vi "State Process.vi"(8 "error in (no error)":errorcluster, 11 "View Model":T1) -> (0 "error out":errorcluster, 3 "View Model":T1)   [LabVIEW 2017]
doc: "Process actual elevator controller state."
uses:
  View Model/Controls/View Model.ctl
  View Model/Controls/Shared Model.ctl
  Error Handler/Controls/Error Model.ctl
  Error Handler/Controls/Error Data.ctl
  Error Handler/Controls/Error Level.ctl
  Configuration/Controls/Config Model.ctl
  Configuration/Controls/Config Data Record.ctl
  Configuration/Controls/Config Command.ctl
  Controls/Control Model.ctl
  Controls/Elevator Location.ctl
  Controls/Elevator Status.ctl
  Controls/Control Event.ctl
  Controls/Control CMD.ctl
  Controls/Controller - Overhead.ctl
  Controls/Timer Commands.ctl
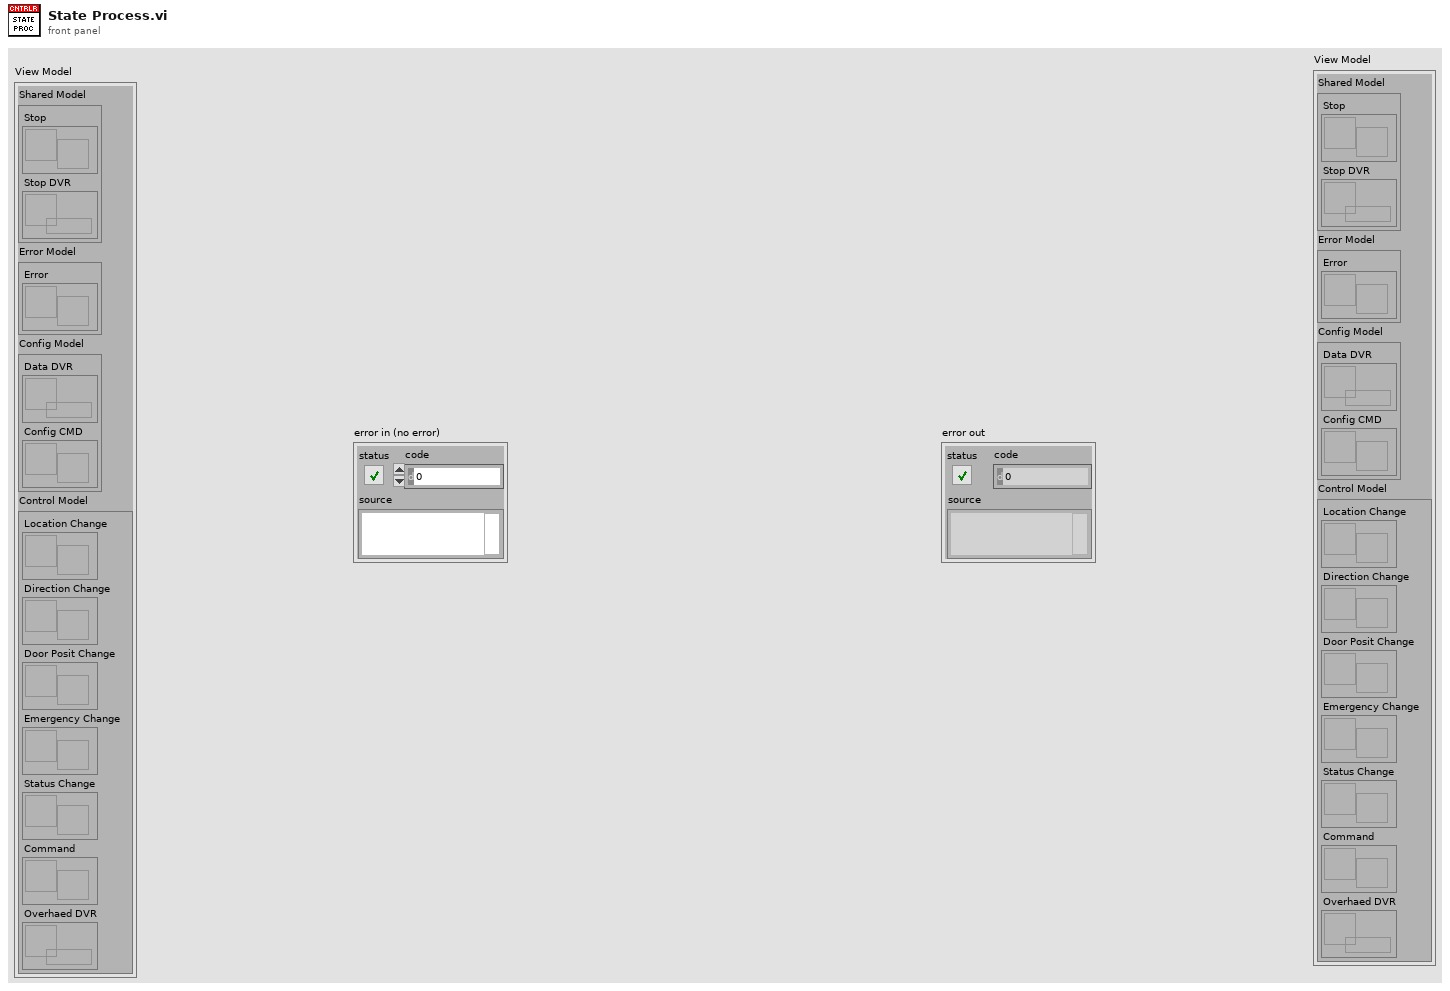
[diagram p1: front panel]
types:
  T1 = typedef "View Model.ctl" = cluster{"Shared Model":T2, "Error Model":T3, "Config Model":T4, "Control Model":T5}
  T2 = typedef "Shared Model.ctl" = cluster{"Stop":refnum<user-event>, "Stop DVR":refnum<data-value>}
  T3 = typedef "Error Model.ctl" = cluster{"Error":refnum<user-event>}
  T4 = typedef "Config Model.ctl" = cluster{"Data DVR":refnum<data-value>, "Config CMD":refnum<user-event>}
  T5 = typedef "Control Model.ctl" = cluster{"Location Change":refnum<user-event>, "Direction Change":refnum<user-event>, "Door Posit Change":refnum<user-event>, "Emergency Change":refnum<user-event>, "Status Change":refnum<user-event>, "Command":refnum<user-event>, "Overhaed DVR":refnum<data-value>}
  T6 = typedef "Elevator Status.ctl" = enum16{"No Request", "Initial", "Wait for 1st Request", "Start and Move", "Continue Move", "Analysis", "Stop at Floor", "Open/Close Door", "Emergency Call", "Terminate"}
  T7 = typedef "Timer Commands.ctl" = enum16{"Start", "Restart", "Get", "Pause"}
  T8 = typedef "Elevator Location.ctl" = enum16{"1st Floor", "2nd Floor", "3rd Floor", "4th Floor"}
  T9 = typedef "Control CMD.ctl" = enum16{"Idle", "Call", "Go Up", "Go Down", "Go to Floor", "Open Door", "Close Door", "Emergency"}
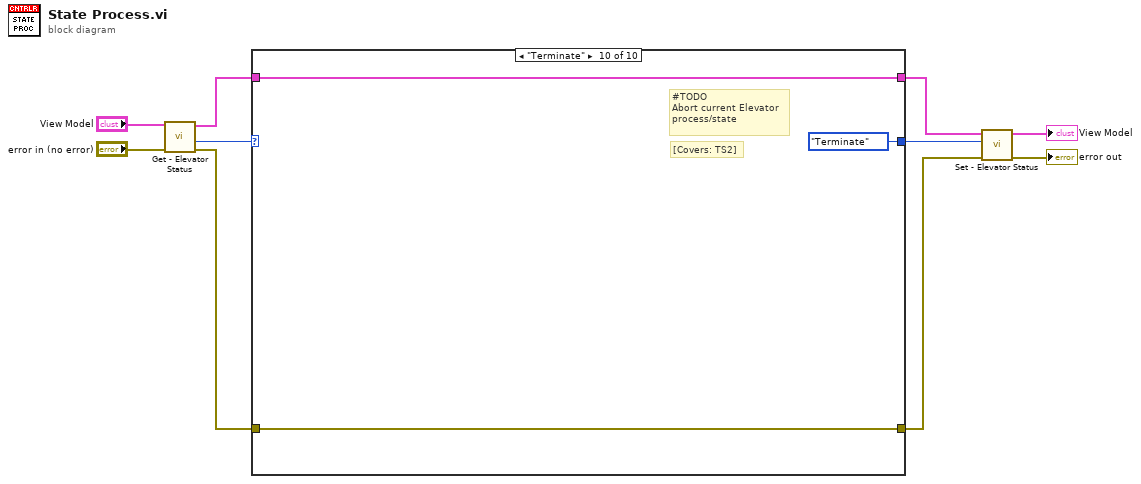
[diagram p0: block diagram]
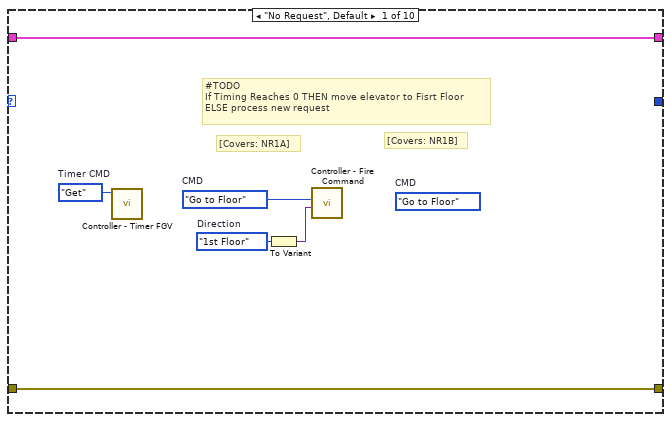
[diagram p2: hidden frame]
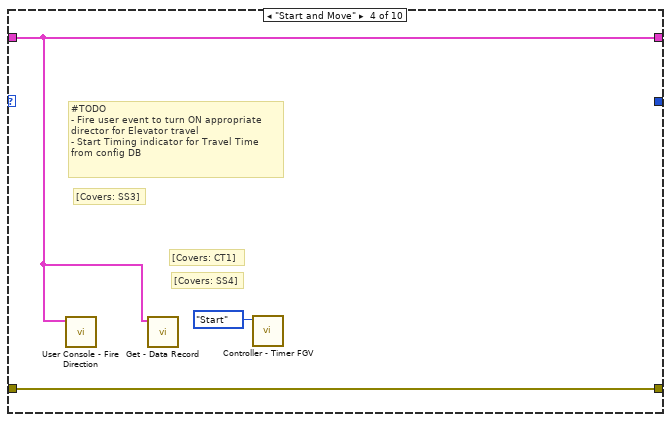
[diagram p5: hidden frame]
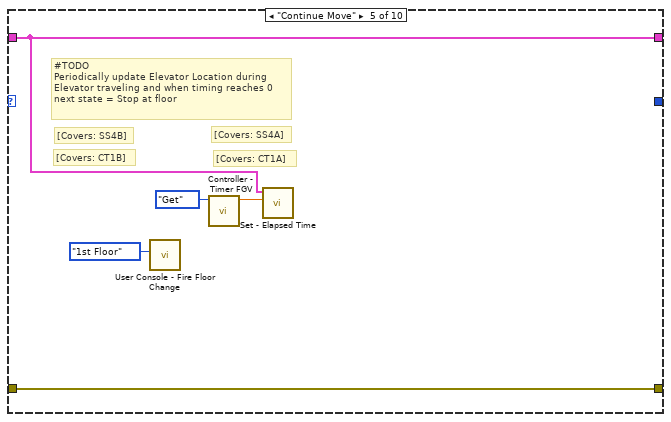
[diagram p6: hidden frame]
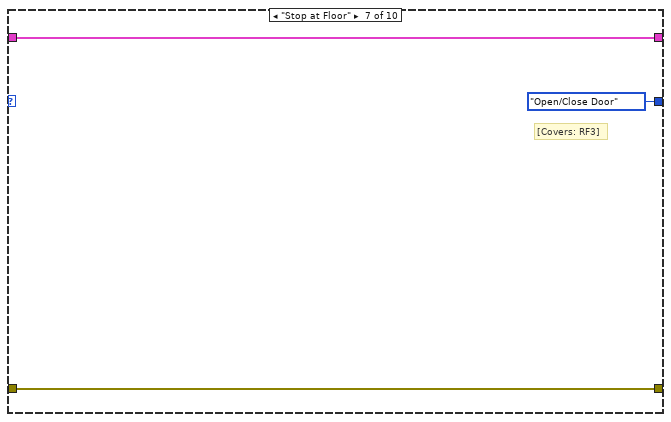
[diagram p8: hidden frame]
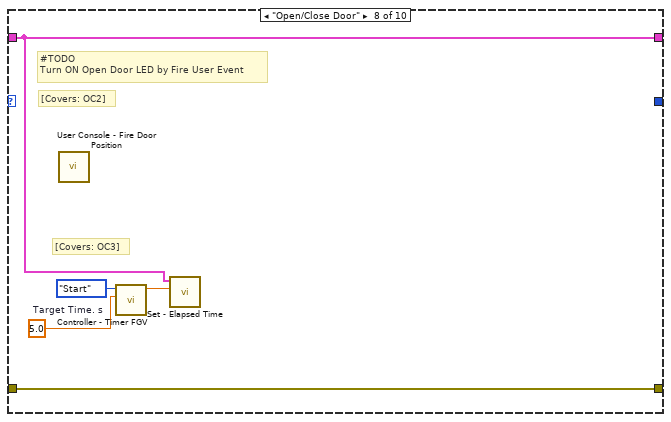
[diagram p9: hidden frame]
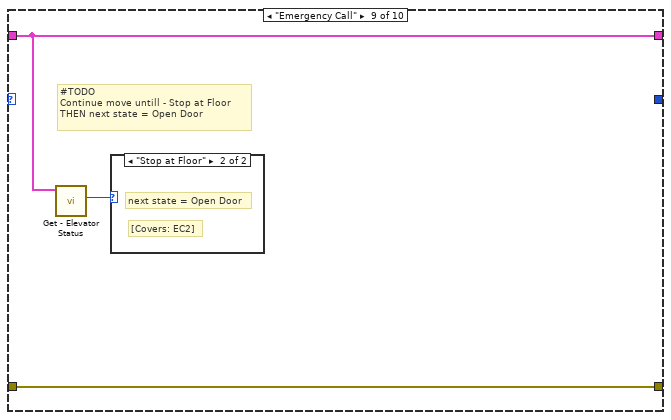
[diagram p10: hidden frame]
diagram:
  n1 = call "Get - Elevator Status.vi"("error in (no error)"="error in (no error)", "View Model"="View Model") -> ("error out"=w2:errorcluster, "Next Status"=w9:T6, "View Model"=w8:T1)  [unwired: 6 in, 1 out]
  n2 = case shown="\"Terminate\"" w9 {
    selector: w9 -> [_ w17 _ _ _ _ _ _ _ _]
    tunnel: w8 -> [w16 w19 w21 w22 w25 w31 w34 w36 w40 w45]
    tunnel: [w16 w19 w21 w22 w25 w31 w34 w36 w40 w45] -> w7
    tunnel: w2 -> [w15 w18 w20 w24 w29 w30 w33 w39 w42 w44]
    tunnel: [w15 w18 w20 w24 w29 w30 w33 w39 w42 w44] -> w3
    tunnel: [_ w17 _ _ _ _ Elevator_Status."Open/Close Door" ("Next Status") _ _ Elevator_Status."Terminate" ("Next Status")] -> w1
    frame "No Request", Default {
      (unwired) Control_CMD."Go to Floor"  # CMD
      w12 = Elevator_Location."1st Floor"  # Direction
      w13 = Control_CMD."Go to Floor"  # CMD
      w14 = Timer_Commands."Get"  # Timer CMD
      # "[Covers: NR1B]"
      # "[Covers: NR1A]"
      # "#TODO\nIf Timing Reaches 0 THEN move elevator to Fisrt Floor\nELSE process new request"
      n3 = call "Controller - Timer FGV.vi"("Timer CMD"=w14) -> ()  [unwired: 8 in, 3 out]
      n4 = To Variant(anything=w12) -> (Variant=w11:variant)
      n5 = call "Controller - Fire Command.vi"("Data"=w11, "CMD"=w13) -> ()  [unwired: 8 in, 2 out]
    }
    frame "Initial" {
    }
    frame "Wait for 1st Request" {
    }
    frame "Start and Move" {
      # "[Covers: CT1]"
      # "[Covers: SS4]"
      # "[Covers: SS3]"
      # "#TODO\n- Fire user event to turn ON appropriate \ndirector for Elevator travel\n- Start Timing indicator for Travel Time\nfrom config DB"
      n6 = call "User Console - Fire Direction.vi"("View Model"=w22) -> ()  [unwired: 9 in, 2 out]
      n7 = call "Get - Data Record.vi"("View Model"=w22) -> ()  [unwired: 8 in, 3 out]
      n8 = call "Controller - Timer FGV.vi"("Timer CMD"=Timer_Commands."Start") -> ()  [unwired: 8 in, 3 out]
    }
    frame "Continue Move" {
      # "[Covers: CT1B]"
      # "[Covers: CT1A]"
      # "[Covers: SS4B]"
      # "[Covers: SS4A]"
      # "#TODO\nPeriodically update Elevator Location during\nElevator traveling and when timing reaches 0\nnext state = Stop at floor"
      n9 = call "User Console - Fire Floor Change.vi"("Floor Selection"=Elevator_Location."1st Floor") -> ()  [unwired: 9 in, 2 out]
      n10 = call "Controller - Timer FGV.vi"("Timer CMD"=Timer_Commands."Get") -> ("Elapsed Time"=w26:dbl)  [unwired: 8 in, 2 out]
      n11 = call "Set - Elapsed Time.vi"("Elapsed Time"=w26, "View Model"=w25) -> ()  [unwired: 8 in, 2 out]
    }
    frame "Analysis" {
      # "[Covers: AS2C]"
      # "[Covers: AS2B]"
      # "[Covers: AS2A]"
      # "[Covers: AS2]"
      # "#TODO\nDetermines next ELevator states based on DVR values.\nIF the Elevator should stop on current floor THEN next state = Stop at Floor\nIF the Elevator should continue travel in current direction \n  THEN next state=Continue Move\nIF the Elevator changes direction THEN next state = Start and Move"
    }
    frame "Stop at Floor" {
      # "[Covers: RF3]"
    }
    frame "Open/Close Door" {
      w35 = 5.0  # Target Time. s
      # "[Covers: OC3]"
      # "[Covers: OC2]"
      # "#TODO\nTurn ON Open Door LED by Fire User Event"
      n12 = call "User Console - Fire Door Position.vi"() -> ()  [unwired: 10 in, 2 out]
      n13 = call "Controller - Timer FGV.vi"("Target Time. s"=w35, "Timer CMD"=Timer_Commands."Start") -> ("Elapsed Time"=w38:dbl)  [unwired: 7 in, 2 out]
      n14 = call "Set - Elapsed Time.vi"("Elapsed Time"=w38, "View Model"=w36) -> ()  [unwired: 8 in, 2 out]
    }
    frame "Emergency Call" {
      # "#TODO\nContinue move untill - Stop at Floor\nTHEN next state = Open Door"
      n15 = call "Get - Elevator Status.vi"("View Model"=w40) -> ("Current Status"=w41:T6)  [unwired: 7 in, 3 out]
      n16 = case shown="\"Stop at Floor\"" w41 {
        frame "Continue Move", Default {
        }
        frame "Stop at Floor" {
          # "[Covers: EC2]"
          # "next state = Open Door"
        }
      }
    }
    frame "Terminate" {
      # "[Covers: TS2]"
      # "#TODO\nAbort current Elevator\nprocess/state"
    }
  }
  n17 = call "Set - Elevator Status.vi"("error in (no error)"=w3, "Current Status"=w1, "View Model"=w7) -> ("error out"=→"error out":errorcluster, "View Model"=→"View Model":T1)  [unwired: 7 in]
